vi "Find Instrument.vi"(10 "Instrument Name":string, 11 "Instrumentes to Use":T1(array[cluster])) -> (2 "Instrument Found?":bool, 3 "Instrument.lvclass":refnum<class "Instrument.lvclass">)   [LabVIEW 2020, in "Test Framework.lvclass"]
uses:
  Test Framework.lvclass
  Instruments/Instrument.lvclass
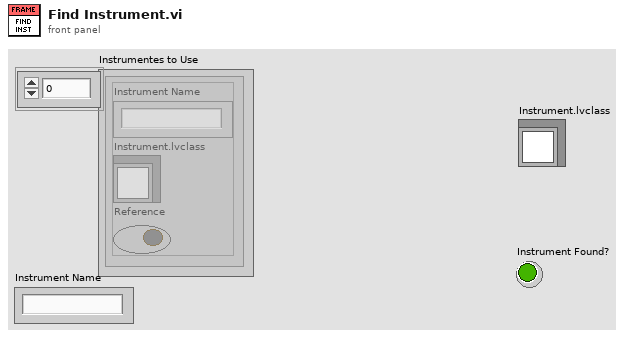
[diagram p1: front panel]
types:
  T1 = cluster{"Instrument Name":string, "Instrument.lvclass":refnum<class "Instrument.lvclass">, "Reference":bool}[]
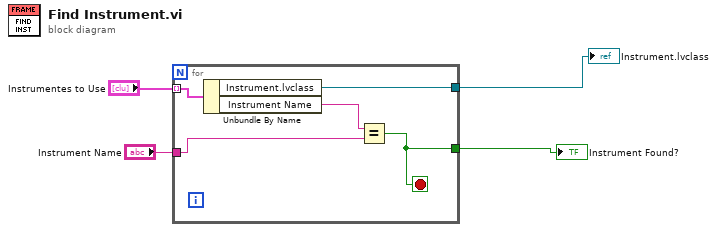
[diagram p0: block diagram]
diagram:
  n1 = for {
    tunnel: "Instrumentes to Use" -> [w9] mode=indexing
    tunnel: "Instrument Name" -> [w7]
    tunnel: [w6] -> w2
    tunnel: [w5] -> w1
    stop <- w6 stop-if-true
    n2 = Unbundle By Name(w9) -> ("Instrument.lvclass"=w5:refnum<class "Instrument.lvclass">, "Instrument Name"=w8:string)
    n3 = Equal?(x=w8, y=w7) -> (x = y?=w6:bool)
  }
  "Instrument Found?" <- w2
  "Instrument.lvclass" <- w1
